vi "ASCII_NUM U8 (SubVI).vi"(1 "String":string) -> (0 "Number":i32)   [LabVIEW 8.6]
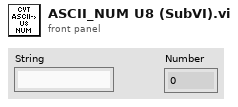
[diagram p1: front panel]
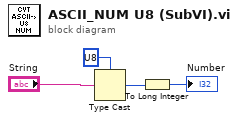
[diagram p0: block diagram]
diagram:
  n1 = Type Cast(type=u8 ?, x="String") -> (*(type *) &x=w3:u8)
  n2 = To Long Integer(number=w3) -> (32bit integer=→"Number":i32)
